vi "Pose2DFuser.vi"(9 "Allowable Error":dbl, 11 "Pose Array":T1[](array[typedef])) -> (3 "Fused Pose":T1)   [LabVIEW 2018]
uses:
  Pose2D.ctl
  40746a38-4c73-4684-bdac-85829db4b9b0.vi
  <vilib>/Array/Sort 2D Array - Pop Stack.vi
  <vilib>/Array/Sort 2D Array - Push Stack.vi
panel:
  out "sorted 2D array":dbl[][](array[numeric])
  out "Total Points Used":dbl
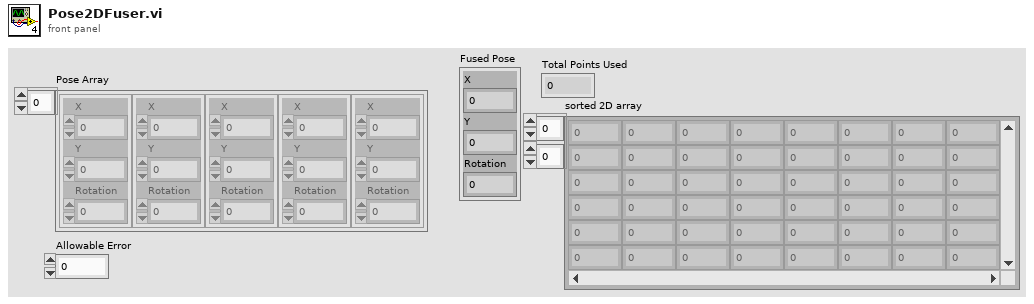
[diagram p1: front panel]
types:
  T1 = typedef "Pose2D.ctl" = cluster{"X":dbl, "Y":dbl, "Rotation":dbl}
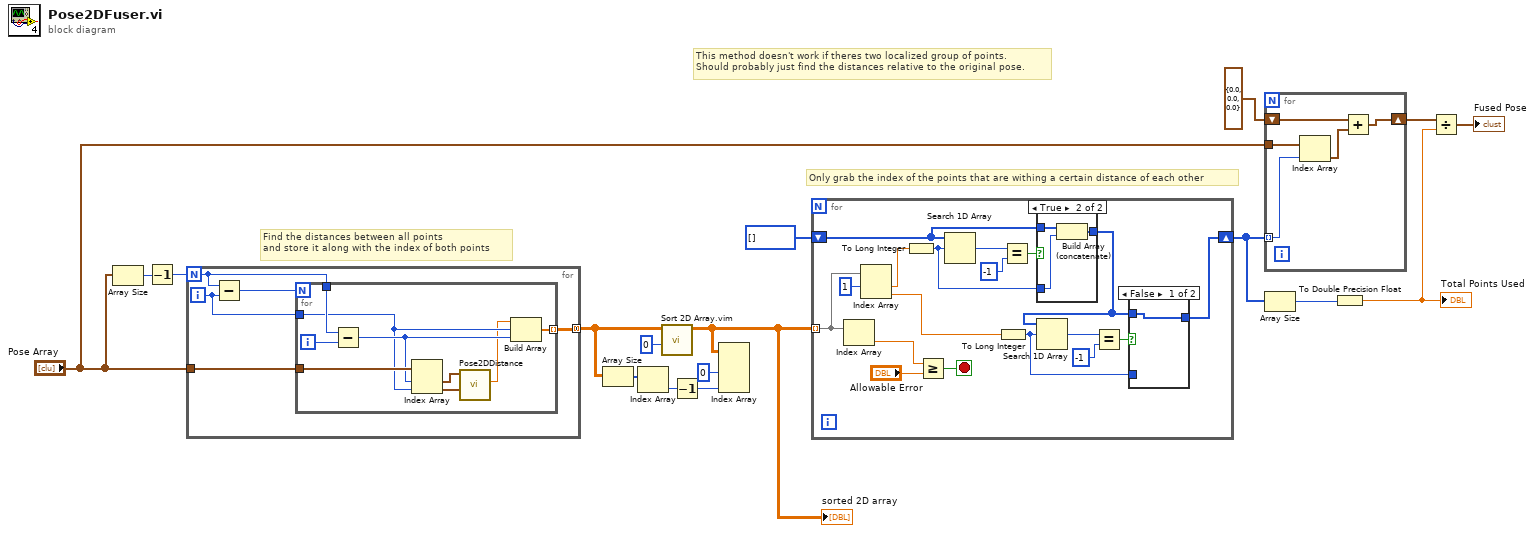
[diagram p0: block diagram]
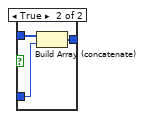
[diagram p2: hidden frame]
diagram:
  # "This method doesn't work if theres two localized group of points.\nShould probably just find the distances relative to the original pose."
  # "Only grab the index of the points that are withing a certain distance of each other"
  # "Find the distances between all points\nand store it along with the index of both points"
  n1 = Array Size(array="Pose Array") -> (size(s)=w16:i32)
  n2 = Decrement(x=w16) -> (x-1=w15:i32)
  n3 = for {
    N: w15 -> [w19]
    tunnel: "Pose Array" -> [w18]
    tunnel: [w21] -> w4 mode=concatenating
    i -> [w22]
    n4 = Subtract(x=w19, y=w22) -> (x-y=w20:i32)
    n5 = for {
      N: w20 -> [_]
      tunnel: w22 -> [w26]
      tunnel: [w31] -> w21 mode=indexing
      tunnel: w19 -> [w30]
      tunnel: w18 -> [w28]
      i -> [w29]
      n6 = Subtract(x=w30, y=w29) -> (x-y=w27:i32)
      n7 = Index Array(array=w28, index #1=w27, index #2=w26) -> (element #1=w25:T1, element #2=w24:T1)
      n8 = call "Pose2DDistance.vi"("Second Pose2D"=w24, "First Pose2D"=w25) -> ("Distance"=w23:dbl)  [unwired: 9 in]
      n9 = Build Array(w23, w26, w27) -> (w31:dbl[])
    }
  }
  n10 = Array Size(array=w4) -> (size(s)=w3:i32[])
  n11 = Index Array(array=w3) -> (element=w2:i32)  [unwired: 1 in]
  n12 = call "Sort 2D Array.vim"("index"=0, "2D array"=w4) -> ("sorted 2D array"=w6:dbl[][])  [unwired: 8 in, 1 out]
  "sorted 2D array" <- w6
  n13 = Decrement(x=w2) -> (x-1=w1:i32)
  n14 = Index Array(array=w6, index (col) #1=0 ("disabled index (col)"), index (col) #2=w1) -> ()  [unwired: 2 in, 2 out]
  n15 = for {
    tunnel: w6 -> [w47] mode=indexing
    shift-right: [w33] -> w11
    shift-left: i32[] [] -> [w41]
    stop <- w48 stop-if-true
    n16 = Index Array(array=w47) -> (element=w49:dbl)  [unwired: 1 in]
    n17 = Index Array(array=w47, index #1=1 ("index")) -> (element #1=w45:dbl, element #2=w34:dbl)  [unwired: 1 in]
    n18 = To Long Integer(number=w45) -> (32bit integer=w40:i32)
    n19 = Greater Or Equal?(x=w49, y="Allowable Error") -> (x >= y?=w48:bool)
    n20 = Search 1D Array(1D array=w41, element=w40) -> (index of element=w44:i32)  [unwired: 1 in]
    n21 = To Long Integer(number=w34) -> (32bit integer=w39:i32)
    n22 = Equal?(x=w44, y=-1) -> (x = y?=w42:bool)
    n23 = case shown="True" w42 {
      tunnel: w41 -> [w54 w57]
      tunnel: w40 -> [_ w56]
      tunnel: [w54 w55] -> w35
      frame False {
      }
      frame True {
        n24 = Build Array (concatenate)(w57, w56) -> (w55:i32[])
      }
    }
    n25 = Search 1D Array(1D array=w35, element=w39) -> (index of element=w36:i32)  [unwired: 1 in]
    n26 = Equal?(x=w36, y=-1) -> (x = y?=w38:bool)
    n27 = case shown="False" w38 {
      tunnel: w35 -> [w50 w53]
      tunnel: w39 -> [_ w52]
      tunnel: [w50 w51] -> w33
      frame False {
      }
      frame True {
        n28 = Build Array (concatenate)(w53, w52) -> (w51:i32[])
      }
    }
  }
  n29 = for {
    tunnel: w11 -> [w61] mode=indexing
    tunnel: "Pose Array" -> [w62]
    shift-right: [w59] -> w12
    shift-left: T1 {"X"=0.0, "Y"=0.0, "Rotation"=0.0} ("Pose2D") -> [w58]
    n30 = Index Array(array=w62, index=w61) -> (element=w60:T1)
    n31 = Add(x=w58, y=w60) -> (x+y=w59:T1)
  }
  n32 = Array Size(array=w11) -> (size(s)=w10:i32)
  n33 = To Double Precision Float(number=w10) -> (double precision float=w7:dbl)
  "Total Points Used" <- w7
  n34 = Divide(x=w12, y=w7) -> (x/y=→"Fused Pose":T1)
